vi "SquareXandY.vi"(11 "Rectangle Descriptor":T1) -> (2 "Numeric":sgl, 3 "Numeric 2":sgl)   [LabVIEW 2021]
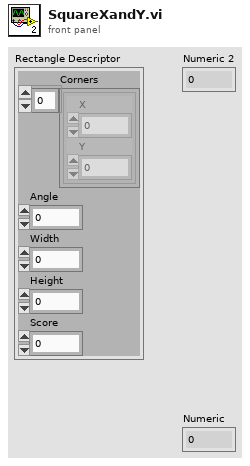
[diagram p1: front panel]
types:
  T1 = cluster{"Corners":cluster{"X":sgl, "Y":sgl}[], "Angle":dbl, "Width":dbl, "Height":dbl, "Score":dbl}
  T2 = cluster{"Corners[0]":cluster{"X":sgl, "Y":sgl}, "Corners[1]":cluster{"X":sgl, "Y":sgl}, "Corners[2]":cluster{"X":sgl, "Y":sgl}, "Corners[3]":cluster{"X":sgl, "Y":sgl}, "Corners[4]":cluster{"X":sgl, "Y":sgl}, "Corners[5]":cluster{"X":sgl, "Y":sgl}, "Corners[6]":cluster{"X":sgl, "Y":sgl}, "Corners[7]":cluster{"X":sgl, "Y":sgl}, "Corners[8]":cluster{"X":sgl, "Y":sgl}}
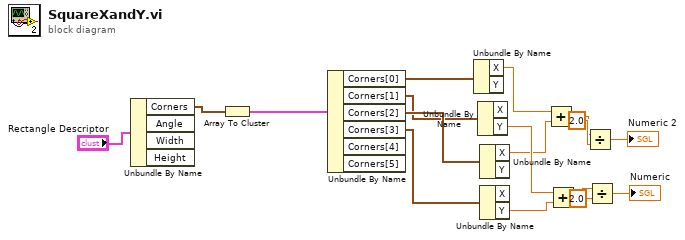
[diagram p0: block diagram]
diagram:
  n1 = Unbundle By Name("Rectangle Descriptor") -> ("Corners"=w2:cluster{"X":sgl, "Y":sgl}[])  [unwired: 3 out]
  n2 = Array To Cluster(array=w2) -> (cluster=w3:T2)
  n3 = Unbundle By Name(w3) -> ("Corners[0]"=w4:cluster{"X":sgl, "Y":sgl}, "Corners[1]"=w5:cluster{"X":sgl, "Y":sgl}, "Corners[2]"=w6:cluster{"X":sgl, "Y":sgl}, "Corners[3]"=w7:cluster{"X":sgl, "Y":sgl})  [unwired: 2 out]
  n4 = Unbundle By Name(w4) -> ("X"=w8:sgl)  [unwired: 1 out]
  n5 = Unbundle By Name(w5) -> ("Y"=w10:sgl)  [unwired: 1 out]
  n6 = Unbundle By Name(w6) -> ("X"=w9:sgl)  [unwired: 1 out]
  n7 = Unbundle By Name(w7) -> ("Y"=w11:sgl)  [unwired: 1 out]
  n8 = Add(x=w8, y=w9) -> (x+y=w12:sgl)
  n9 = Add(x=w10, y=w11) -> (x+y=w14:sgl)
  n10 = Divide(x=w12, y=sgl 2.0) -> (x/y=→"Numeric 2":sgl)
  n11 = Divide(x=w14, y=sgl 2.0) -> (x/y=→"Numeric":sgl)
